vi "has_GUI.vi"(8 "error in (no error)":errorcluster, 11 "DL090629NoiseTraceProcessor in":refnum<class "TraceProcessorDL090629Noise.lvclass">) -> (0 "error out":errorcluster, 2 "has GUI?":bool, 3 "DL090629NoiseTraceProcessor out":refnum<class "TraceProcessorDL090629Noise.lvclass">)   [LabVIEW 2010, in "TraceProcessorDL090629Noise.lvclass"]
uses:
  TraceProcessorDL090629Noise.lvclass
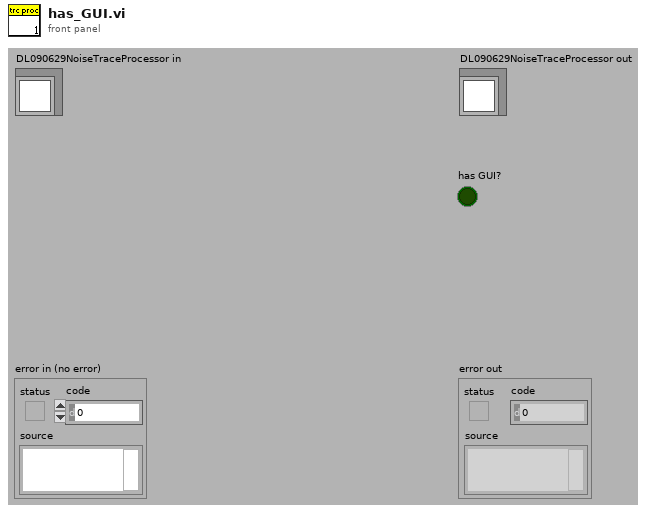
[diagram p1: front panel]
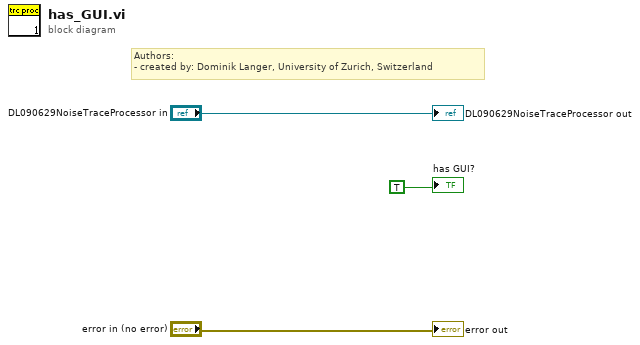
[diagram p0: block diagram]
diagram:
  # "Authors: \n- created by: Dominik Langer, University of Zurich, Switzerland"
  "error out" <- "error in (no error)"
  "DL090629NoiseTraceProcessor out" <- "DL090629NoiseTraceProcessor in"
  "has GUI?" <- TRUE
